vi "FPGA_DIOReadFilterSelect.vi"(8 "error in (no error)":errorcluster, 10 "channel index":u8, 11 "DIODeviceRef In":T1) -> (0 "error out":errorcluster, 2 "FilterSelect":u8, 3 "DIODeviceRef Out":T1)   [LabVIEW 2017]
uses:
  <vilib>/Rock Robotics/SystemInterfaces/DIO/FPGA_DIODevRef.ctl
  <vilib>/Rock Robotics/SystemInterfaces/System/FPGA_SystemFPGA Ref Global.vi
  <vilib>/Utility/error.llb/Error Cluster From Error Code.vi
  <vilib>/rvi/errors/niLvFpgaAdjustHostInterfaceError.vi
  <vilib>/rvi/interface/nirviReadWriteControl/nirviReadWriteControl.xnode
  <vilib>/Rock Robotics/SystemInterfaces/System/FPGA_SystemFRC FPGA Ref.ctl
  NiFpgaLv.dll
  <vilib>/rvi/interface/Simulation/niFpgaSimulationCallBeginRW.vi
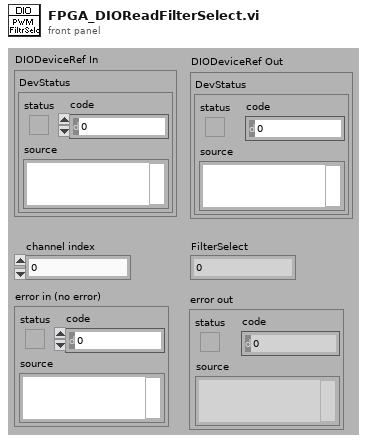
[diagram p1: front panel]
types:
  T1 = typedef "FPGA_DIODevRef.ctl" = cluster{"DevStatus":errorcluster}
  T2 = typedef "FPGA_SystemFRC FPGA Ref.ctl" = refnum<k20>
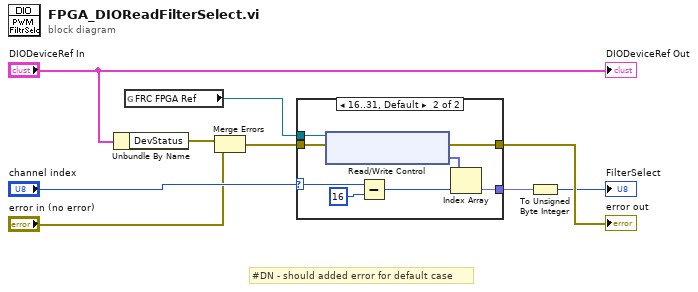
[diagram p0: block diagram]
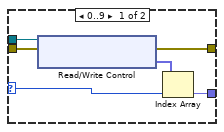
[diagram p2: hidden frame]
diagram:
  # "#DN - should added error for default case"
  n1 = Unbundle By Name("DIODeviceRef In") -> ("DevStatus"=w4:errorcluster)
  n2 = global read "FPGA_SystemFPGA Ref Global.vi" "FRC FPGA Ref"() -> (w5:T2)
  n3 = Merge Errors(w4, "error in (no error)") -> (w3:errorcluster)
  n4 = case shown="16..31, Default" "channel index" {
    selector: "channel index" -> [w10 w18]
    tunnel: [w15 w23] -> w9
    tunnel: [w14 w22] -> w6
    tunnel: w3 -> [w13 w21]
    tunnel: w5 -> [w12 w20]
    frame 0..9 {
      n5 = xnode "Read/Write Control"("FPGA VI Reference In"=w12, "error in"=w13) -> ("error out"=w15:errorcluster, "DIO.FilterSelectHdr"=w11:fxp<+,2,2>[])  [unwired: 1 out]
      n6 = Index Array(array=w11, index=w10) -> (element=w14:fxp<+,2,2>)
    }
    frame 16..31, Default {
      n7 = xnode "Read/Write Control"("FPGA VI Reference In"=w20, "error in"=w21) -> ("error out"=w23:errorcluster, "DIO.FilterSelectMXP"=w19:fxp<+,2,2>[])  [unwired: 1 out]
      n8 = Subtract(x=w18, y=u8 16) -> (x-y=w17:u8)
      n9 = Index Array(array=w19, index=w17) -> (element=w22:fxp<+,2,2>)
    }
  }
  "error out" <- w9
  n10 = To Unsigned Byte Integer(number=w6) -> (unsigned 8bit integer=→"FilterSelect":u8)
  "DIODeviceRef Out" <- "DIODeviceRef In"
